vi "Write Exception Status.vi"(8 "error in":errorcluster, 10 "exception status":u8 format="%02x", 11 "device data model in":refnum<class "Standard Data Model.lvclass">) -> (0 "error out":errorcluster, 3 "device data model out":refnum<class "Standard Data Model.lvclass">)   [LabVIEW 2012, in "Standard Data Model.lvclass"]
doc: "Sets the exception status in the device data model."
uses:
  Standard Data Model.lvclass
  Standard Data Model.lvclass/Standard Data Model.ctl
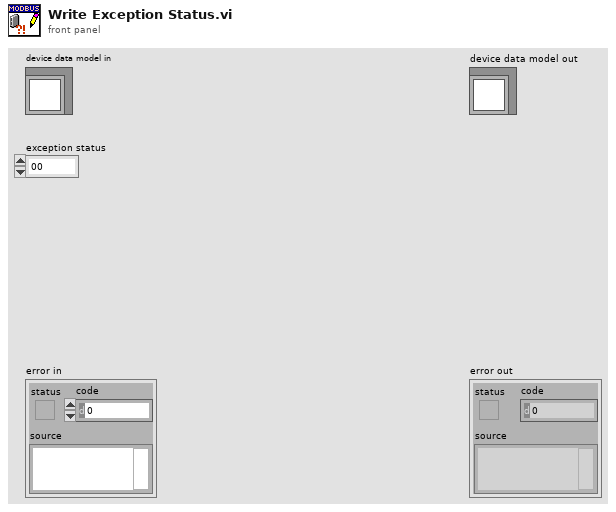
[diagram p1: front panel]
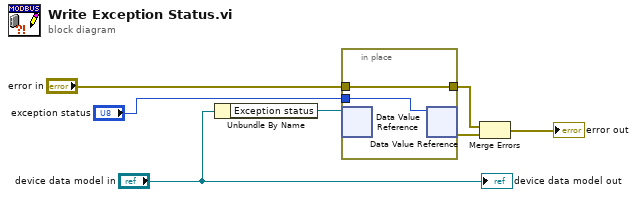
[diagram p0: block diagram]
diagram:
  n1 = Unbundle By Name("device data model in") -> ("Exception status"=w4:refnum<data-value>)
  n2 = in-place {
    in-place-border: "error in" -> [w9]
    in-place-border: [w9] -> w2
    in-place-border: "exception status" -> [w8]
    n3 = in-place-dvr #1(w4) -> ()  [unwired: 2 out]
    n4 = in-place-dvr #1(w8) -> (w3:errorcluster)  [unwired: 1 out]
  }
  n5 = Merge Errors(w2, w3) -> (→"error out":errorcluster)
  "device data model out" <- "device data model in"
